vi "Memory.Pointer.Parameter Check.Subset.vi"(7 "calling vi name":string, 8 "error in (no error)":errorcluster, 9 "length":u64 format="%d bytes", 10 "offset":u64 format="%d bytes", 11 "Pointer in":refnum<class "Memory.Pointer.Void.lvclass">) -> (0 "error out":errorcluster, 1 "length out":u64 format="%d bytes", 2 "offset out":u64 format="%d bytes", 3 "Pointer out":refnum<class "Memory.Pointer.Void.lvclass">)   [LabVIEW 2016, in "Memory.Pointer.Void.lvclass"]
uses:
  Memory.Pointer.Void.lvclass
  Typedefs/Memory.Pointer.Parameters.ctl
  Pointer/Memory.Pointer.lvclass
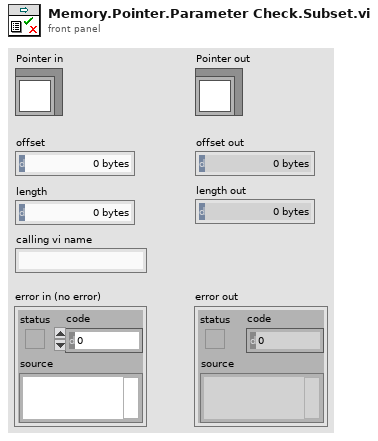
[diagram p1: front panel]
types:
  T1 = typedef "Memory.Pointer.Void.lvclass/Memory.Pointer.Parameters.ctl" = enum16{"offset", "length", "size", "subset"}
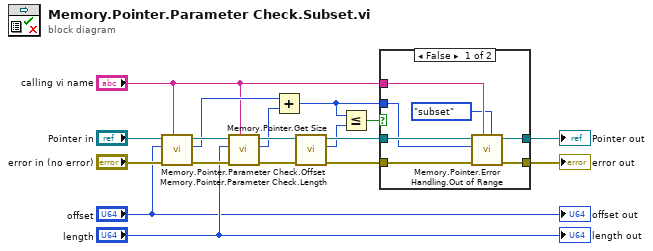
[diagram p0: block diagram]
diagram:
  n1 = call "Memory.Pointer.Parameter Check.Offset.vi"("calling vi name"="calling vi name", "error in (no error)"="error in (no error)", "offset"="offset", "Pointer in"="Pointer in") -> ("error out"=w12:errorcluster, "offset out"=w10:u64, "Pointer out"=w13:refnum<class "Memory.Pointer.Void.lvclass">)  [unwired: 5 in]
  n2 = call "Memory.Pointer.Parameter Check.Length.vi"("calling vi name"="calling vi name", "error in (no error)"=w12, "length"="length", "Pointer in"=w13) -> ("error out"=w17:errorcluster, "length out"=w16:u64, "Pointer out"=w18:refnum<class "Memory.Pointer.Void.lvclass">)  [unwired: 5 in]
  n3 = Add(x=w10, y=w16) -> (x+y=w3:u64)
  n4 = call "Memory.Pointer.Get Size.vi"("error in (no error)"=w17, "Pointer in"=w18) -> ("error out"=w8:errorcluster, "size"=w4:u64, "Pointer out"=w5:refnum<class "Memory.Pointer.Void.lvclass">)  [unwired: 7 in]
  n5 = Less Or Equal?(x=w3, y=w4) -> (x <= y?=w1:bool)
  n6 = case shown="False" w1 {
    tunnel: [w25 w27] -> w7
    tunnel: w8 -> [w24 w27]
    tunnel: w3 -> [w20 _]
    tunnel: w5 -> [w23 w26]
    tunnel: [w22 w26] -> w6
    tunnel: "calling vi name" -> [w21 _]
    frame False {
      n7 = call "Memory.Pointer.Error Handling.Out of Range.vi"("parameter"=Memory.Pointer.Parameters."subset", "source vi name"=w21, "error in (no error)"=w24, "value"=w20, "pointer in"=w23) -> ("error out"=w25:errorcluster, "pointer out"=w22:refnum<class "Memory.Pointer.lvclass">)  [unwired: 5 in]
    }
    frame True {
    }
  }
  "error out" <- w7
  "Pointer out" <- w6
  "length out" <- "length"
  "offset out" <- "offset"
